vi "LoadSubPanel.vi"(4 "MainProgQEvent":refnum<user-event>, 6 "MainProgQ":refnum<queue>, 8 "error in (no err)":errorcluster caption="entrée d'erreur (pas d'erreur)", 9 "PanelIndex":i32[](array[numeric]), 10 "SubPanel Refs":refnum<vi>[](array[refnum]), 11 "LoadedInst":refnum<class "BaseDevice.lvclass">[](array[class])) -> (0 "sortie d'erreur":errorcluster, 3 "LoadedInst Out":refnum<class "BaseDevice.lvclass">[](array[class]) caption="LoadedInst")   [LabVIEW 2019, in "BaseDevice.lvclass"]
uses:
  BaseDevice.lvclass
  BaseDevice.lvclass/BaseDevice.ctl
  ClassQueueMess.ctl
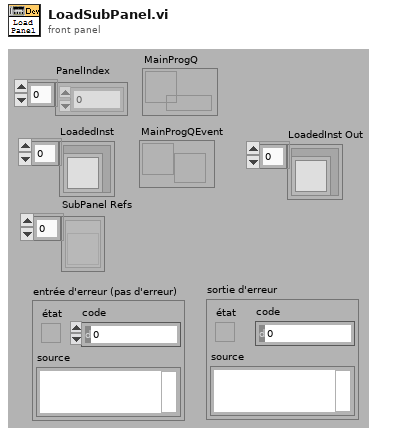
[diagram p1: front panel]
types:
  T1 = typedef "ClassQueueMess.ctl" = u16
  T2 = typedef "LVPointTypeDef.ctl" = cluster{"Horizontal":i16, "Vertical":i16}
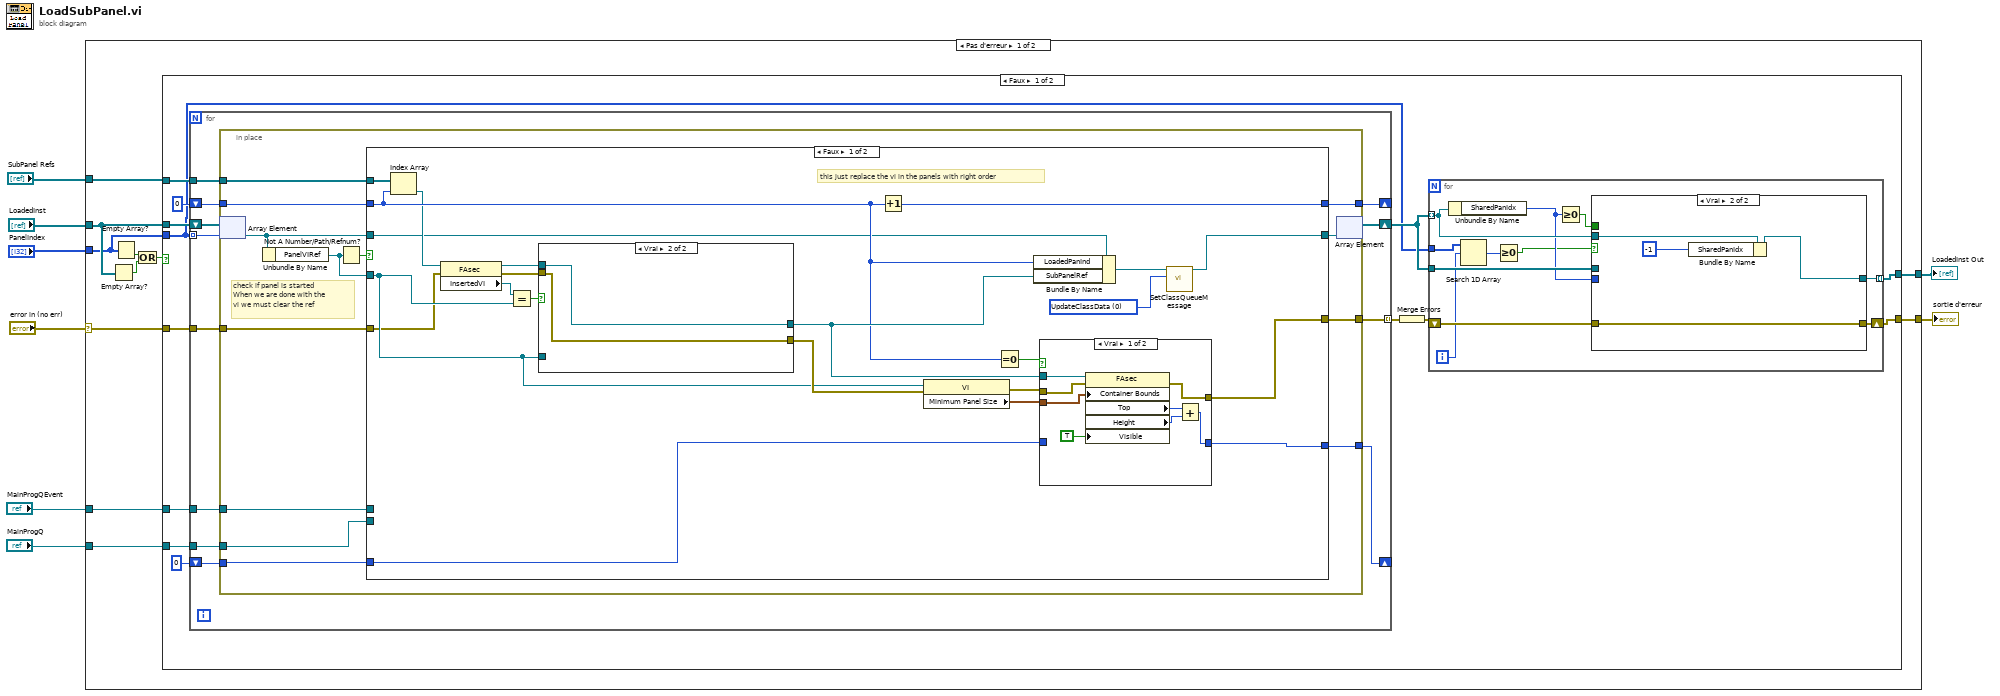
[diagram p0: block diagram]
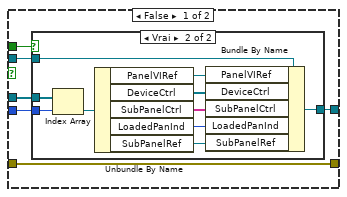
[diagram p2: hidden frame]
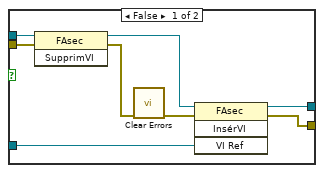
[diagram p4: hidden frame]
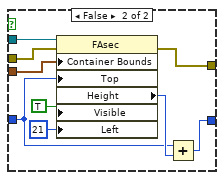
[diagram p5: hidden frame]
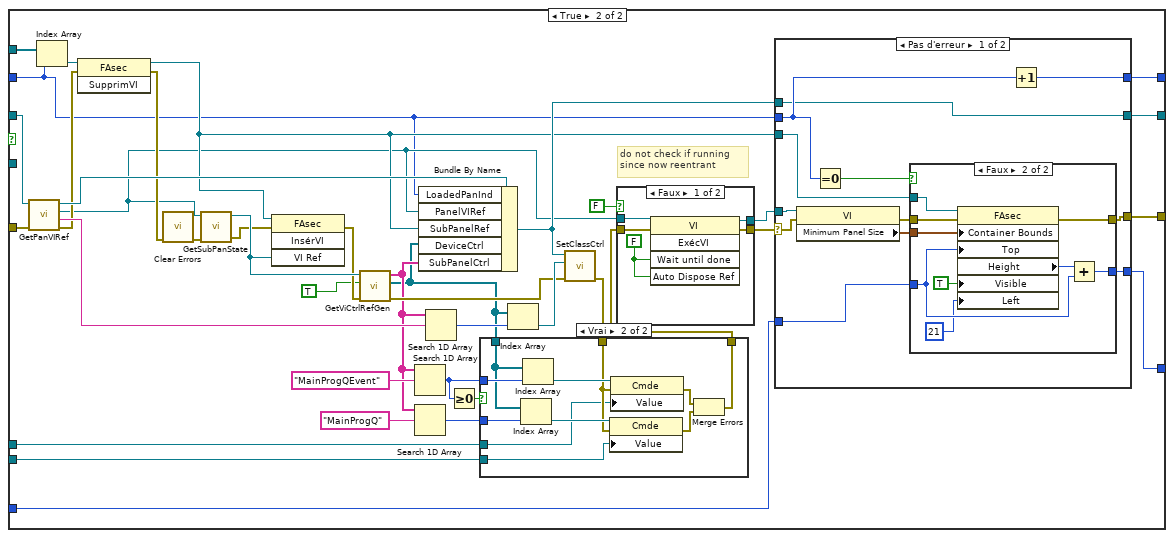
[diagram p6: hidden frame]
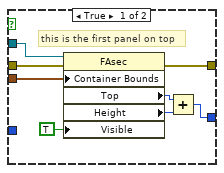
[diagram p9: hidden frame]
diagram:
  n1 = case shown="Pas d'erreur" "error in (no err)" {
    selector: "error in (no err)" -> [w19 w232]
    tunnel: "SubPanel Refs" -> [w18 _]
    tunnel: [w17 w232] -> w7
    tunnel: [w16 w233] -> w5
    tunnel: "LoadedInst" -> [w15 w233]
    tunnel: "PanelIndex" -> [w9 _]
    tunnel: "MainProgQEvent" -> [w11 _]
    tunnel: "MainProgQ" -> [w10 _]
    frame No Error {
      n2 = Empty Array?(array=w15) -> (empty?=w13:bool)
      n3 = Empty Array?(array=w9) -> (empty?=w12:bool)
      n4 = Or(x=w12, y=w13) -> (x .or. y?=w14:bool)
      n5 = case shown="Faux" w14 {
        tunnel: w19 -> [w32 w230]
        tunnel: w18 -> [w30 _]
        tunnel: w15 -> [w29 w231]
        tunnel: [w23 w230] -> w17
        tunnel: [w21 w231] -> w16
        tunnel: w9 -> [w20 _]
        tunnel: w11 -> [w26 _]
        tunnel: w10 -> [w25 _]
        frame False {
          n6 = for {
            tunnel: w32 -> [w76]
            tunnel: [w75] -> w31 mode=indexing
            tunnel: w30 -> [w74]
            shift-right: [w72] -> _
            shift-left: 0 -> [w73]
            shift-right: [w71] -> _
            shift-left: u32 0 -> [w70]
            tunnel: w20 -> [w69] mode=indexing
            shift-right: [w68] -> w22
            shift-left: w29 -> [w67]
            tunnel: w26 -> [w66]
            tunnel: w25 -> [w65]
            n7 = in-place {
              in-place-border: w76 -> [w82]
              in-place-border: [w89] -> w75
              in-place-border: w74 -> [w88]
              in-place-border: w73 -> [w87]
              in-place-border: [w86] -> w72
              in-place-border: [w85] -> w71
              in-place-border: w70 -> [w84]
              in-place-border: w66 -> [w78]
              in-place-border: w65 -> [w77]
              # "check if panel is started\nWhen we are done with the\nvi we must clear the ref"
              n8 = in-place-array #1(w67, w69) -> (w81:refnum<class "BaseDevice.lvclass">)
              n9 = Unbundle By Name(w81) -> ("PanelVIRef"=w79:refnum<vi>)
              n10 = Not A Number/Path/Refnum?(number/path/refnum=w79) -> (NaN/Path/Refnum?=w80:bool)
              n11 = case shown="Faux" w80 {
                tunnel: [w109 w139] -> w89
                tunnel: w88 -> [w108 w177]
                tunnel: w87 -> [w102 w140]
                tunnel: [w111 w176] -> w86
                tunnel: [w106 w175] -> w85
                tunnel: w84 -> [w107 w150]
                tunnel: [w91 w171] -> w83
                tunnel: w82 -> [w95 w168]
                tunnel: w81 -> [w96 w167]
                tunnel: w79 -> [w100 _]
                tunnel: w78 -> [_ w145]
                tunnel: w77 -> [_ w144]
                frame False {
                  w90 = T1 0 items=["UpdateClassData", "UpdateMainClass", "UpdateDataBind", "ReInitDevice"] ("Menu déroulant")
                  # "this just replace the vi in the panels with right order"
                  n12 = Index Array(array=w108, index=w102) -> (element=w99:refnum<vi>)
                  n13 = property class="FAsec"(reference=w99, error in=w95) -> (reference out=w98:refnum<vi>, error out=w94:errorcluster, "InsertedVI"=w97:refnum<vi>)
                  n14 = Equal?(x=w97, y=w100) -> (x = y?=w93:bool)
                  n15 = case shown="Vrai" w93 {
                    tunnel: w94 -> [w119 w121]
                    tunnel: [w116 w121] -> w104
                    tunnel: [w115 w120] -> w103
                    tunnel: w100 -> [w113 _]
                    tunnel: w98 -> [w112 w120]
                    frame False {
                      n16 = invoke on="Nœud de méthode" class="FAsec" method="SupprimVI"(reference=w112, error in=w119) -> (reference out=w118:refnum<vi>, error out=w117:errorcluster)  [unwired: 1 in, 1 out]
                      n17 = call <vilib>:"Clear Errors.vi"("error in (no error)"=w117) -> ("error out"=w114:errorcluster)  [unwired: 5 in, 1 out]
                      n18 = invoke on="Nœud de méthode" class="FAsec" method="InsérVI"(reference=w118, error in=w114, "VI Ref"=w113) -> (reference out=w115:refnum<vi>, error out=w116:errorcluster)  [unwired: 1 in, 2 out]
                    }
                    frame True {
                    }
                  }
                  n19 = Increment(x=w102) -> (x+1=w111:i32)
                  n20 = property class="VI"(reference=w100, error in=w104) -> (error out=w105:errorcluster, "Minimum Panel Size"=w101:T2)  [unwired: 1 out]
                  n21 = Equal To 0?(x=w102) -> (x = 0?=w110:bool)
                  n22 = Bundle By Name(cluster=w96, "LoadedPanInd"=w102, "SubPanelRef"=w103) -> (w92:refnum<class "BaseDevice.lvclass">)
                  n23 = case shown="Vrai" w110 {
                    tunnel: w105 -> [w129 w138]
                    tunnel: w103 -> [w128 w137]
                    tunnel: [w127 w136] -> w109
                    tunnel: [w125 w135] -> w106
                    tunnel: w107 -> [_ w131]
                    tunnel: w101 -> [w122 w134]
                    frame True {
                      n24 = property class="FAsec"(reference=w128, error in=w129, "Container Bounds"=w122, "Visible"=TRUE) -> (error out=w127:errorcluster, "Top"=w126:i32, "Height"=w124:u32)  [unwired: 1 out]
                      n25 = Add(x=w126, y=w124) -> (x+y=w125:u32)
                    }
                    frame False {
                      n26 = property class="FAsec"(reference=w137, error in=w138, "Container Bounds"=w134, "Top"=w131, "Visible"=TRUE, "Left"=21 ("Position:Gauche")) -> (error out=w136:errorcluster, "Height"=w132:u32)  [unwired: 1 out]
                      n27 = Add(x=w131, y=w132) -> (x+y=w135:u32)
                    }
                  }
                  n28 = call-dynamic "SetClassQueueMessage.vi"("Menu déroulant"=w90, "BaseDevice.lvclass"=w92) -> ("BaseDevice.lvclass Out"=w91:refnum<class "BaseDevice.lvclass">)  [unwired: 8 in, 1 out]
                }
                frame True {
                  # "do not check if running \nsince now reentrant"
                  n29 = call "GetPanVIRef.vi"("error in (no error)"=w168, "BaseDevice en entrée"=w167) -> ("error out"=w165:errorcluster, "ClassName"=w169:string, "PanelVIRef"=w141:refnum<vi>, "BaseDevice en sortie"=w170:refnum<class "BaseDevice.lvclass">)  [unwired: 6 in]
                  n30 = Index Array(array=w177, index=w140) -> (element=w166:refnum<vi>)
                  n31 = invoke on="Nœud de méthode" class="FAsec" method="SupprimVI"(reference=w166, error in=w165) -> (reference out=w142:refnum<vi>, error out=w164:errorcluster)  [unwired: 1 in, 1 out]
                  n32 = call <vilib>:"Clear Errors.vi"("error in (no error)"=w164) -> ("error out"=w163:errorcluster)  [unwired: 5 in, 1 out]
                  n33 = call "GetSubPanState.vi"("ErrorIn(No Error)"=w163, "référence"=w141) -> ("sortie d'erreur"=w161:errorcluster, "Ref_Out"=w162:refnum<vi>)  [unwired: 6 in, 2 out]
                  n34 = invoke on="Nœud de méthode" class="FAsec" method="InsérVI"(reference=w142, error in=w161, "VI Ref"=w162) -> (error out=w160:errorcluster)  [unwired: 1 in, 3 out]
                  n35 = call <userlib>:"GetViCtrlRefGen.vi"("ErrorIn(No Error)"=w160, "InclTabCTrl"=TRUE, "VIRef"=w162) -> ("sortie d'erreur"=w157:errorcluster, "ControlsRefs"=w151:refnum<vi>[], "ControlsNames"=w152:string[])  [unwired: 6 in]
                  n36 = Search 1D Array(1D array=w152, element="MainProgQEvent" ("élément")) -> (index of element=w149:i32)  [unwired: 1 in]
                  n37 = Search 1D Array(1D array=w152, element="MainProgQ" ("élément")) -> (index of element=w154:i32)  [unwired: 1 in]
                  n38 = Bundle By Name(cluster=w170, "LoadedPanInd"=w140, "PanelVIRef"=w141, "SubPanelRef"=w142, "DeviceCtrl"=w151, "SubPanelCtrl"=w152) -> (w159:refnum<class "BaseDevice.lvclass">)
                  n39 = Search 1D Array(1D array=w152, element=w169) -> (index of element=w172:i32)  [unwired: 1 in]
                  n40 = Greater Or Equal To 0?(x=w149) -> (x >= 0?=w148:bool)
                  n41 = Index Array(array=w151, index=w172) -> (element=w158:refnum<vi>)
                  n42 = call-dynamic "SetClassCtrl.vi"("error in (no error)"=w157, "ClassCtrlRef"=w158, "BaseDevice en entrée"=w159) -> ("error out"=w147:errorcluster)  [unwired: 7 in, 1 out]
                  n43 = case shown="Vrai" w148 {
                    tunnel: w149 -> [_ w189]
                    tunnel: w154 -> [_ w188]
                    tunnel: w151 -> [_ w187]
                    tunnel: w147 -> [w178 w184]
                    tunnel: [w178 w181] -> w146
                    tunnel: w145 -> [_ w180]
                    tunnel: w144 -> [_ w179]
                    frame False {
                    }
                    frame True {
                      n44 = Index Array(array=w187, index=w188) -> (element=w185:refnum<vi>)
                      n45 = Index Array(array=w187, index=w189) -> (element=w186:refnum<vi>)
                      n46 = property class="Cmde"(reference=w185, error in=w184, "Value"=w179) -> (error out=w182:errorcluster)  [unwired: 1 out]
                      n47 = property class="Cmde"(reference=w186, error in=w184, "Value"=w180) -> (error out=w183:errorcluster)  [unwired: 1 out]
                      n48 = Merge Errors(w183, w182) -> (w181:errorcluster)
                    }
                  }
                  n49 = case shown="Faux" FALSE {
                    tunnel: [w194 w195] -> w174
                    tunnel: [w193 w196] -> w173
                    tunnel: w141 -> [w190 w196]
                    tunnel: w146 -> [w191 w195]
                    frame False {
                      w192 = FALSE ("Attendre la fin")
                      n50 = invoke class="VI" method="ExécVI"(reference=w190, error in=w191, "Wait until done"=w192, "Auto Dispose Ref"=w192) -> (reference out=w193:refnum<vi>, error out=w194:errorcluster)  [unwired: 1 in, 3 out]
                    }
                    frame True {
                      # "alreasdy running"
                    }
                  }
                  n51 = case shown="Pas d'erreur" w174 {
                    selector: w174 -> [w204 w228]
                    tunnel: w159 -> [w197 w229]
                    tunnel: [w197 w229] -> w171
                    tunnel: [w202 w228] -> w139
                    tunnel: w142 -> [w205 _]
                    tunnel: w173 -> [w203 _]
                    tunnel: w140 -> [w200 w227]
                    tunnel: [w208 w227] -> w176
                    tunnel: [w201 w226] -> w175
                    tunnel: w150 -> [w198 w226]
                    frame No Error {
                      n52 = property class="VI"(reference=w203, error in=w204) -> (error out=w206:errorcluster, "Minimum Panel Size"=w207:T2)  [unwired: 1 out]
                      n53 = Equal To 0?(x=w200) -> (x = 0?=w199:bool)
                      n54 = case shown="Faux" w199 {
                        tunnel: w207 -> [w216 w225]
                        tunnel: w206 -> [w215 w224]
                        tunnel: w205 -> [w214 w223]
                        tunnel: [w213 w222] -> w202
                        tunnel: [w210 w221] -> w201
                        tunnel: w198 -> [_ w218]
                        frame True {
                          # "this is the first panel on top"
                          n55 = property class="FAsec"(reference=w214, error in=w215, "Container Bounds"=w216, "Visible"=TRUE) -> (error out=w213:errorcluster, "Top"=w211:i32, "Height"=w212:u32)  [unwired: 1 out]
                          n56 = Add(x=w211, y=w212) -> (x+y=w210:u32)
                        }
                        frame False {
                          n57 = property class="FAsec"(reference=w223, error in=w224, "Container Bounds"=w225, "Top"=w218, "Visible"=TRUE, "Left"=21 ("Position:Gauche")) -> (error out=w222:errorcluster, "Height"=w219:u32)  [unwired: 1 out]
                          n58 = Add(x=w219, y=w218) -> (x+y=w221:u32)
                        }
                      }
                      n59 = Increment(x=w200) -> (x+1=w208:i32)
                    }
                    frame Error {
                    }
                  }
                }
              }
              n60 = in-place-array #1(w83) -> (w68:refnum<class "BaseDevice.lvclass">[])  [unwired: 1 out]
            }
          }
          n61 = Merge Errors(w31) -> (w24:errorcluster)
          n62 = for {
            tunnel: w22 -> [w41] mode=indexing
            shift-right: [w38] -> w23
            shift-left: w24 -> [w43]
            tunnel: w22 -> [w40]
            tunnel: [w42] -> w21 mode=indexing
            tunnel: w20 -> [w36]
            i -> [w35]
            n63 = Unbundle By Name(w41) -> ("SharedPanIdx"=w39:i32)
            n64 = Search 1D Array(1D array=w36, element=w35) -> (index of element=w34:i32)  [unwired: 1 in]
            n65 = Greater Or Equal To 0?(x=w34) -> (x >= 0?=w33:bool)
            n66 = Greater Or Equal To 0?(x=w39) -> (x >= 0?=w37:bool)
            n67 = case shown="Vrai" w33 {
              tunnel: w43 -> [w47 w61]
              tunnel: [w45 w63] -> w42
              tunnel: w41 -> [w46 w64]
              tunnel: w40 -> [w49 _]
              tunnel: w39 -> [w48 _]
              tunnel: [w47 w61] -> w38
              tunnel: w37 -> [w44 _]
              frame False {
                n68 = case shown="Vrai" w44 {
                  tunnel: w49 -> [_ w60]
                  tunnel: w48 -> [_ w59]
                  tunnel: w46 -> [w50 w57]
                  tunnel: [w50 w51] -> w45
                  frame False {
                  }
                  frame True {
                    n69 = Index Array(array=w60, index=w59) -> (element=w58:refnum<class "BaseDevice.lvclass">)
                    n70 = Unbundle By Name(w58) -> ("PanelVIRef"=w52:refnum<vi>, "DeviceCtrl"=w53:refnum<vi>[], "SubPanelCtrl"=w55:string[], "LoadedPanInd"=w56:i32, "SubPanelRef"=w54:refnum<vi>)
                    n71 = Bundle By Name(cluster=w57, "PanelVIRef"=w52, "DeviceCtrl"=w53, "SubPanelCtrl"=w55, "LoadedPanInd"=w56, "SubPanelRef"=w54) -> (w51:refnum<class "BaseDevice.lvclass">)
                  }
                }
              }
              frame True {
                n72 = Bundle By Name(cluster=w64, "SharedPanIdx"=-1) -> (w63:refnum<class "BaseDevice.lvclass">)
              }
            }
          }
        }
        frame True {
        }
      }
    }
    frame Error {
    }
  }
  "sortie d'erreur" <- w7
  "LoadedInst Out" <- w5
